vi "Lezeti_Power_Monitor_34_g.vi"() -> ()   [LabVIEW 2014]
uses:
  <vilib>/measure/madcrms.llb/Basic Averaged DC-RMS for N Chan.vi
  <vilib>/measure/madcrms.llb/Basic Averaged DC-RMS for 1 Chan.vi
  <vilib>/Utility/file.llb/Write To Spreadsheet File (DBL).vi
  <vilib>/measure/NI_MAPro.lvlib
panel:
  out "error out":errorcluster
  out "DC Current (Amps)":dbl
  out "DC Voltage":dbl
  out "DC Power (Watts)":dbl
  out "Power Factor":dbl
  in  "Average Power Output File":path
  out "Run Date":string
  out "Run Time":string
  out "Elapsed Time (s)":dbl
  out "Apparent Power (VA)":dbl
  out "Average AC Power (Watts)":dbl
  out "Instantaneous AC Power Waveform":waveform(dbl)[](graph)
  out "RMS Voltage L1-L2":dbl
  out "L1 RMS Current":dbl
  in  "Burden Resistor (ohms) (1000)":dbl
  in  "CT Ratio (Iout/Iin) (.0003332)":dbl
  in  "Acquire Sample Size (1000)":dbl
  in  "Acquire Rate (Hz) (1000)":dbl
  in  "Acquire Timeout (1000)":dbl
  out "AC Line 1 Current Waveform":waveform(dbl)[](graph)
  out "AC Voltage L1-L2":waveform(dbl)[](graph)
  in  "stop":bool
  # "For Lezeti Air Conditioning System (Greenpath Tech)\nBy Matsu Thornton\nJuly 2016"
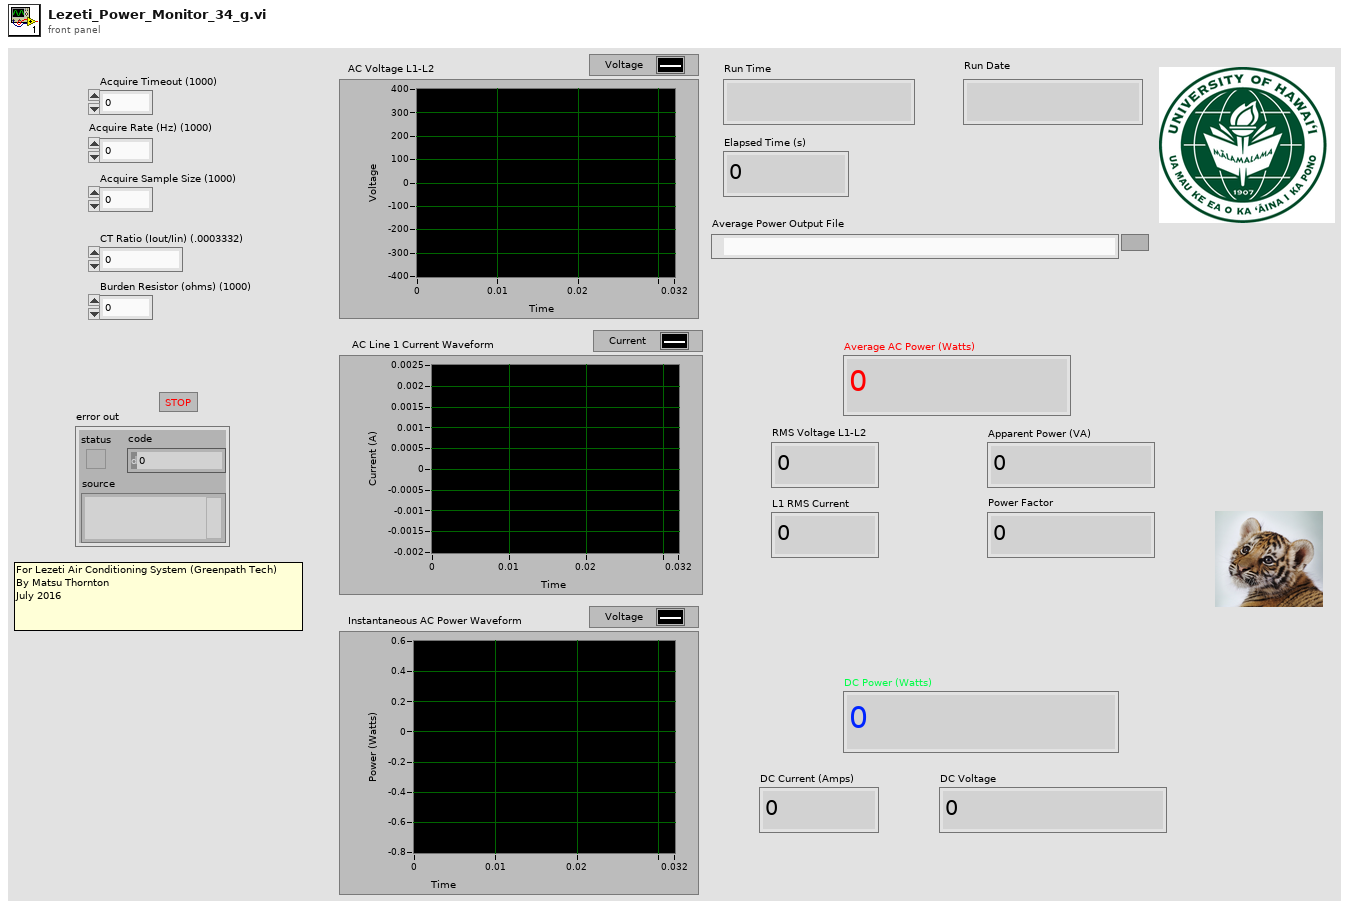
[diagram p1: front panel]
types:
  T1 = typedef "NI_Matrix.lvlib/RealMatrix.ctl" = dbl[][]
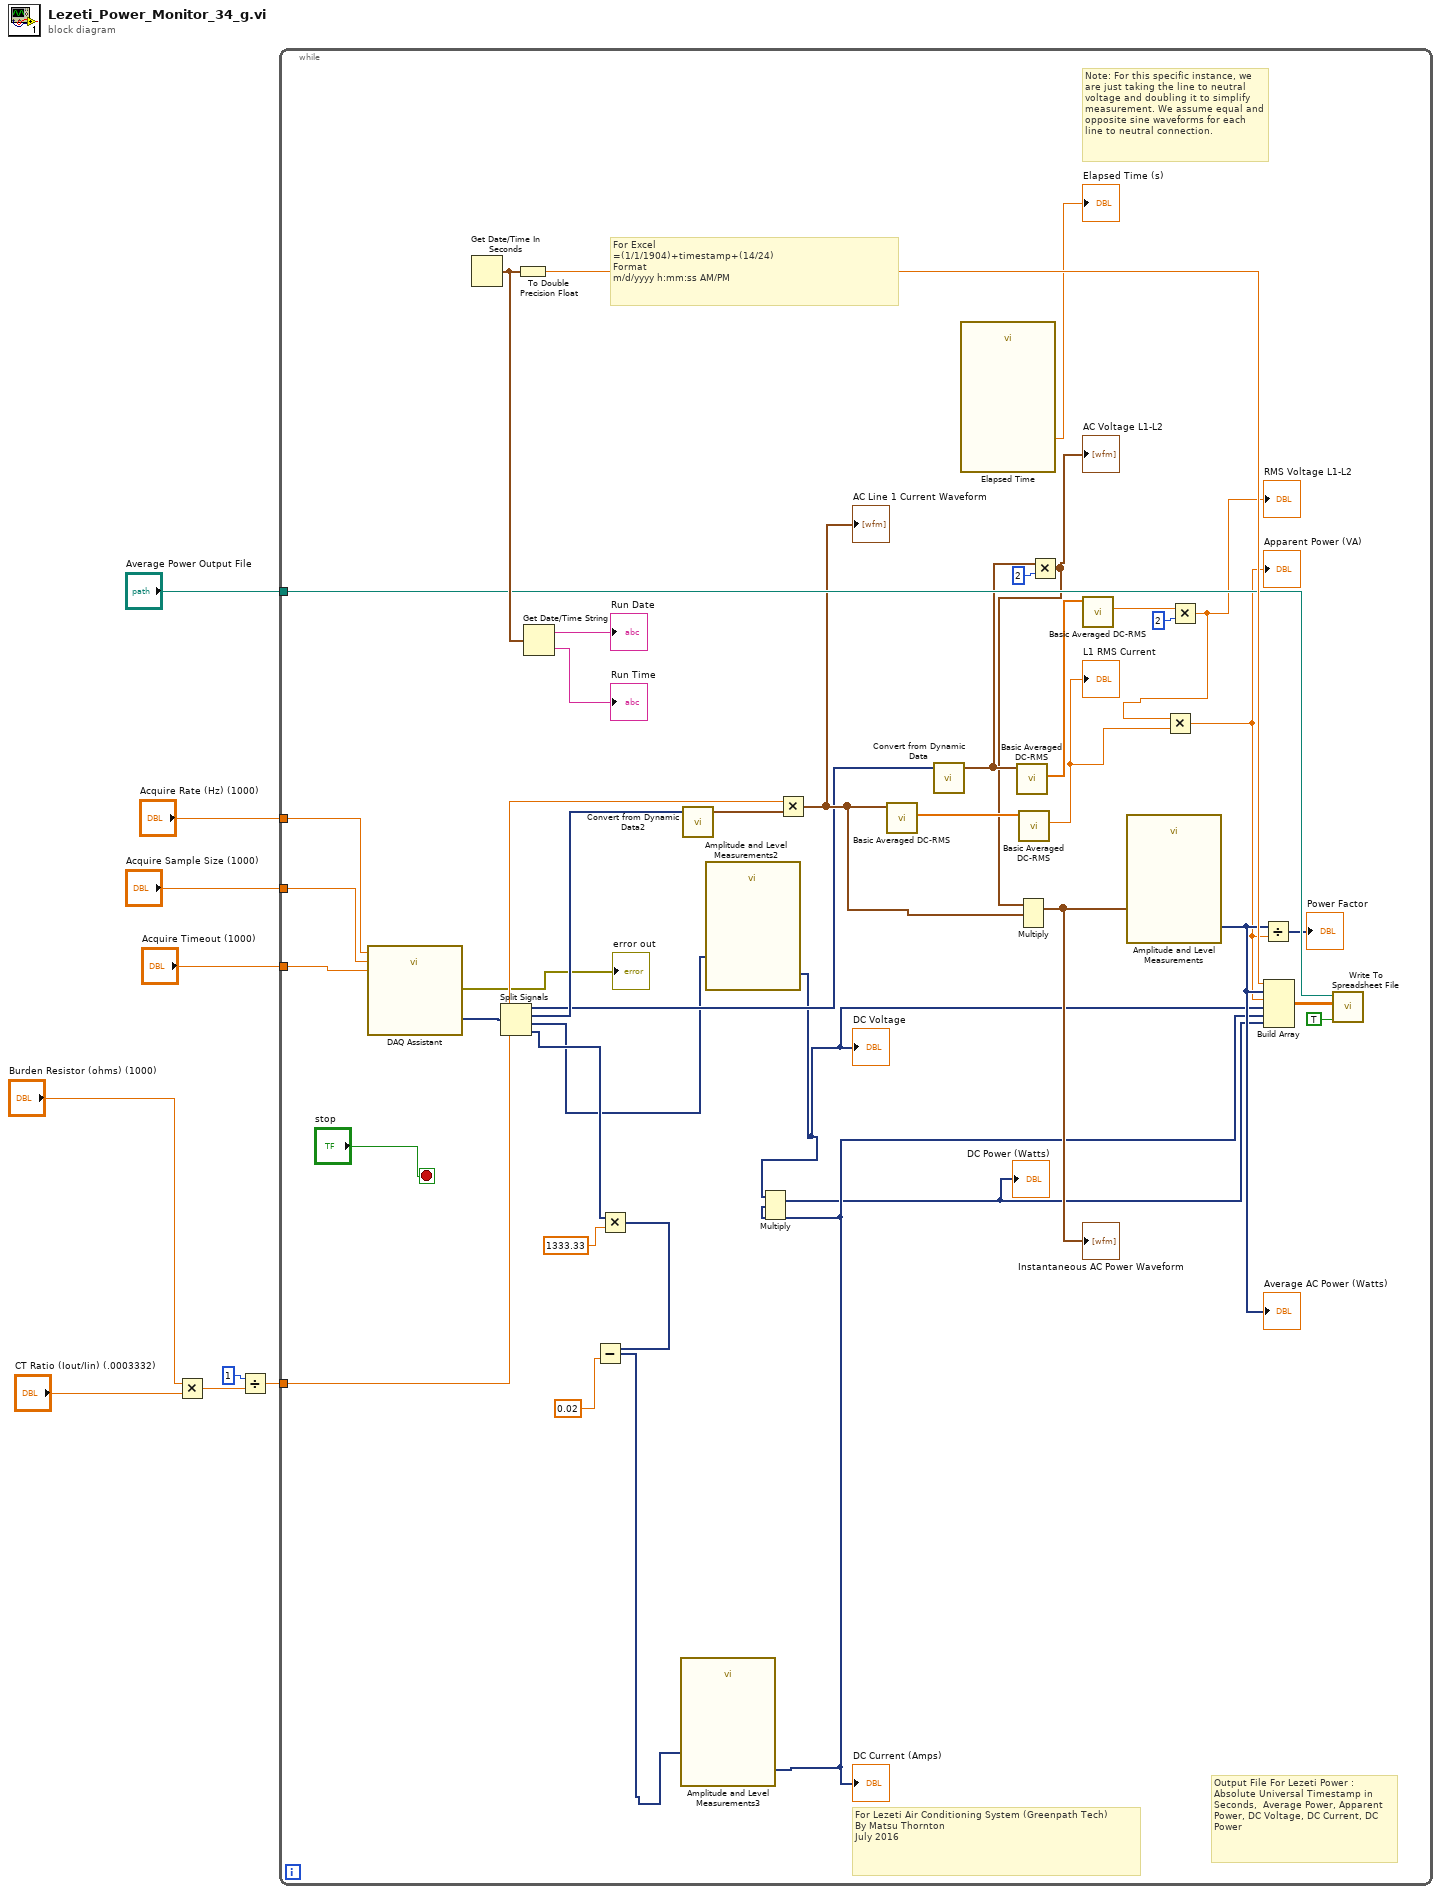
[diagram p0: block diagram]
diagram:
  n1 = Multiply(x="Burden Resistor (ohms) (1000)", y="CT Ratio (Iout/Iin) (.0003332)") -> (x*y=w3:dbl)
  n2 = Divide(x=1, y=w3) -> (x/y=w2:dbl)
  n3 = while {
    tunnel: "Acquire Timeout (1000)" -> [w19]
    tunnel: "Acquire Rate (Hz) (1000)" -> [w21]
    tunnel: "Acquire Sample Size (1000)" -> [w20]
    tunnel: w2 -> [w29]
    tunnel: "Average Power Output File" -> [w39]
    stop <- "stop" stop-if-true
    # "Output File For Lezeti Power :\nAbsolute Universal Timestamp in Seconds,  Average Power, Apparent Power, DC Voltage, DC Current, DC Power"
    # "Note: For this specific instance, we are just taking the line to neutral voltage and doubling it to simplify measurement. We assume equal and opposite sine waveforms for each line to neutral connection."
    # "For Excel\n=(1/1/1904)+timestamp+(14/24)\nFormat\nm/d/yyyy h:mm:ss AM/PM"
    # "For Lezeti Air Conditioning System (Greenpath Tech)\nBy Matsu Thornton\nJuly 2016"
    n4 = call "DAQ Assistant"("rate"=w21, "number of samples"=w20, "timeout (s)"=w19) -> ("data"=w31:dynamicdata, "error out"=→"error out":errorcluster)  [unwired: 13 in, 2 out]
    n5 = Get Date/Time In Seconds() -> (seconds since 1Jan1904=w43:timestamp)
    n6 = Split Signals(w31) -> (w23:dynamicdata, w30:dynamicdata, w15:dynamicdata, w16:dynamicdata)  [unwired: 4 in]
    n7 = To Double Precision Float(number=w43) -> (double precision float=w44:dbl)
    n8 = Get Date/Time String(seconds (now)=w43) -> (date string=→"Run Date":string, time string=→"Run Time":string)  [unwired: 2 in]
    n9 = Multiply(x=w16, y=1333.33) -> (x*y=w12:dynamicdata)
    n10 = Subtract(x=w12, y=0.02) -> (x-y=w10:dynamicdata)
    n11 = call "Amplitude and Level Measurements3"("Signals"=w10) -> ("Mean (DC)"=w28:dynamicdata)  [unwired: 13 in, 1 out]
    "DC Current (Amps)" <- w28
    n12 = call "Convert from Dynamic Data2"("Dynamic Data Type"=w30) -> ("Array of Waveform"=w48:waveform(dbl)[])  [unwired: 3 in]
    n13 = call "Amplitude and Level Measurements2"("Signals"=w15) -> ("Mean (DC)"=w17:dynamicdata)  [unwired: 13 in, 1 out]
    "DC Voltage" <- w17
    n14 = Multiply(1:w28, 2:w17) -> (0:w27:dynamicdata)  [unwired: 1 in, 1 out]
    "DC Power (Watts)" <- w27
    n15 = Multiply(x=w29, y=w48) -> (x*y=w26:waveform(dbl)[])
    "AC Line 1 Current Waveform" <- w26
    n16 = call-poly <vilib>:"Basic Averaged DC-RMS.vi"("signals in"=w26) -> ("RMS values"=w49:dbl[])  [unwired: 7 in, 3 out]
    n17 = call "Convert from Dynamic Data"("Dynamic Data Type"=w23) -> ("Array of Waveform"=w32:waveform(dbl)[])  [unwired: 3 in]
    n18 = call "Elapsed Time"() -> ("Elapsed Time (s)"=→"Elapsed Time (s)":dbl)  [unwired: 12 in, 7 out]
    n19 = call-poly <vilib>:"Basic Averaged DC-RMS.vi"("signals in"=w32) -> ("RMS values"=w50:dbl[])  [unwired: 7 in, 3 out]
    n20 = call-poly <vilib>:"Basic Averaged DC-RMS.vi"("signal in"=w49) -> ("RMS value"=w25:dbl)  [unwired: 7 in, 3 out]
    "L1 RMS Current" <- w25
    n21 = Multiply(x=w32, y=2) -> (x*y=w22:waveform(dbl)[])
    "AC Voltage L1-L2" <- w22
    n22 = Multiply(1:w26, 2:w22) -> (0:w47:waveform(dbl)[])  [unwired: 1 in, 1 out]
    "Instantaneous AC Power Waveform" <- w47
    n23 = call-poly <vilib>:"Basic Averaged DC-RMS.vi"("signal in"=w50) -> ("RMS value"=w34:dbl)  [unwired: 7 in, 3 out]
    n24 = call "Amplitude and Level Measurements"("Signals"=w47) -> ("Mean (DC)"=w38:dynamicdata)  [unwired: 13 in, 1 out]
    "Average AC Power (Watts)" <- w38
    n25 = Multiply(x=w34, y=2) -> (x*y=w24:dbl)
    "RMS Voltage L1-L2" <- w24
    n26 = Multiply(x=w24, y=w25) -> (x*y=w36:dbl)
    "Apparent Power (VA)" <- w36
    n27 = Divide(x=w38, y=w36) -> (x/y=→"Power Factor":dynamicdata)
    n28 = Build Array(w44, w38, w36, w17, w28, w27) -> (w45:T1)
    n29 = call-poly <vilib>:"Write To Spreadsheet File.vi"("append to file? (new file:F)"=TRUE, "2D data"=w45, "file path (dialog if empty)"=w39) -> ()  [unwired: 5 in, 1 out]
  }
